vi "Tokens to String.vi"(8 "error in (no error)":errorcluster, 9 "start index":i32, 11 "Value Tokens":cluster{"Token Type":T1, "Token Value":string}[](array[cluster])) -> (0 "error out":errorcluster, 1 "next index":i32, 3 "String Value":string)   [LabVIEW 2015, in "LVJSON.lvlib" / "JSON String.lvclass"]
uses:
  JSON Data Classes/JSON String/JSON String.lvclass
  Token Types.ctl
  LVJSON.lvlib
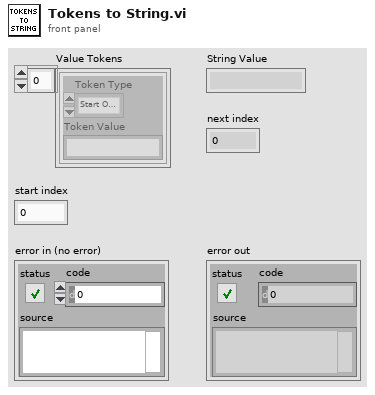
[diagram p1: front panel]
types:
  T1 = typedef "LVJSON.lvlib/Token Types.ctl" = enum32{"Start Object", "End Object", "Start Array", "End Array", "Quotation", "Numeric", "true", "false", "null", "Escape", "Undefined"}
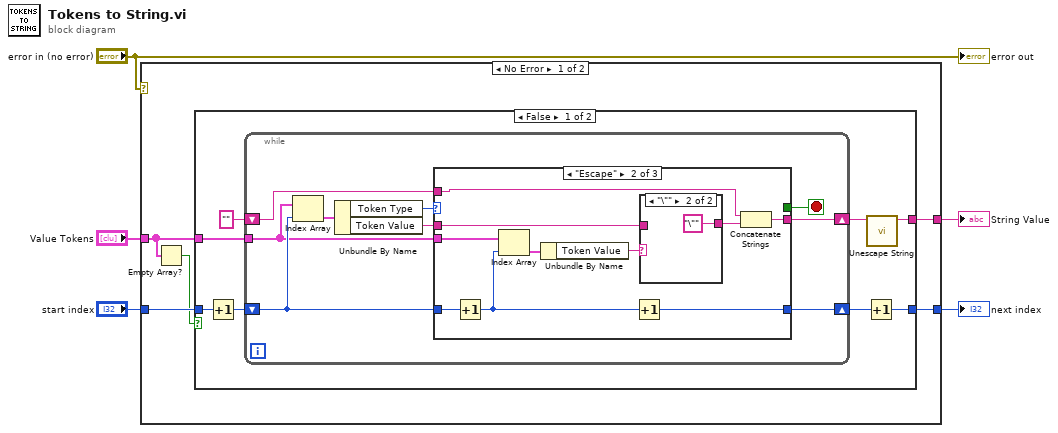
[diagram p0: block diagram]
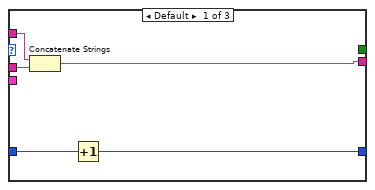
[diagram p2: hidden frame]
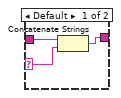
[diagram p3: hidden frame]
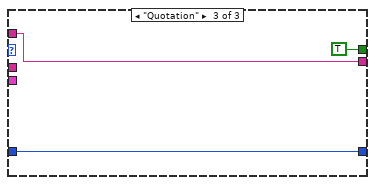
[diagram p4: hidden frame]
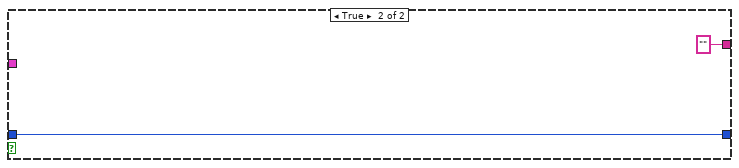
[diagram p5: hidden frame]
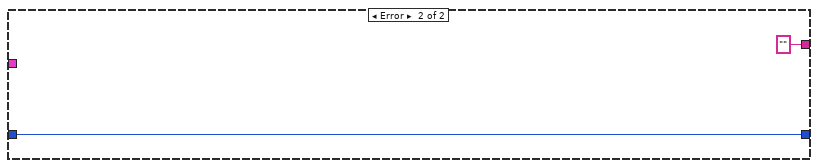
[diagram p6: hidden frame]
diagram:
  n1 = case shown="No Error" "error in (no error)" {
    tunnel: [w10 "" ("Token Value")] -> w5
    tunnel: [w9 w53] -> w1
    tunnel: "start index" -> [w8 w53]
    tunnel: "Value Tokens" -> [w7 _]
    frame No Error {
      n2 = Empty Array?(array=w7) -> (empty?=w6:bool)
      n3 = case shown="False" w6 {
        tunnel: [w11 "" ("Token Value")] -> w10
        tunnel: [w13 w51] -> w9
        tunnel: w8 -> [w15 w51]
        tunnel: w7 -> [w14 _]
        frame False {
          n4 = Increment(x=w15) -> (x+1=w16:i32)
          n5 = while {
            tunnel: w14 -> [w19]
            shift-right: [w21] -> w17
            shift-left: w16 -> [w22]
            shift-right: [w24] -> w12
            shift-left: "" ("Token Value") -> [w20]
            stop <- w26 stop-if-true
            n6 = Index Array(array=w19, index=w22) -> (element=w23:cluster{"Token Type":T1, "Token Value":string})
            n7 = Unbundle By Name(w23) -> ("Token Type"=w27:T1, "Token Value"=w25:string)
            n8 = case shown="\"Escape\"" w27 {
              tunnel: [_ _ TRUE] -> w26
              tunnel: w20 -> [w32 w40 w48]
              tunnel: w25 -> [w31 w35 _]
              tunnel: [w30 w39 w48] -> w24
              tunnel: w22 -> [w29 w42 w47]
              tunnel: [w28 w34 w47] -> w21
              tunnel: w19 -> [_ w41 _]
              frame Default {
                n9 = Concatenate Strings(w32, w31) -> (w30:string)
                n10 = Increment(x=w29) -> (x+1=w28:i32)
              }
              frame "Escape" {
                n11 = Increment(x=w42) -> (x+1=w33:i32)
                n12 = Index Array(array=w41, index=w33) -> (element=w38:cluster{"Token Type":T1, "Token Value":string})
                n13 = Unbundle By Name(w38) -> ("Token Value"=w37:string)
                n14 = Increment(x=w33) -> (x+1=w34:i32)
                n15 = case shown="\"\\\"\"" w37 {
                  selector: w37 -> [w44 _]
                  tunnel: [w43 "\""] -> w36
                  tunnel: w35 -> [w45 _]
                  frame Default {
                    n16 = Concatenate Strings(w45, w44) -> (w43:string)
                  }
                  frame "\"" {
                  }
                }
                n17 = Concatenate Strings(w40, w36) -> (w39:string)
              }
              frame "Quotation" {
              }
            }
          }
          n18 = Increment(x=w17) -> (x+1=w13:i32)
          n19 = call "Unescape String.vi"("value"=w12) -> ("unescaped string"=w11:string)  [unwired: 10 in]
        }
        frame True {
        }
      }
    }
    frame Error {
    }
  }
  "String Value" <- w5
  "next index" <- w1
  "error out" <- "error in (no error)"
